vi "promień_krzywizny_pionowy.vi"(3 "e^2":dbl, 4 "a":dbl, 5 "fi[rad]":dbl) -> (1 "Promien krzywizny równoleżnika":dbl)   [LabVIEW 2015, in "Biblioteka moduł map v3.lvlib" / "Konwersja wsp.lvlib" / "UTM.lvlib"]
uses:
  UTM.lvlib
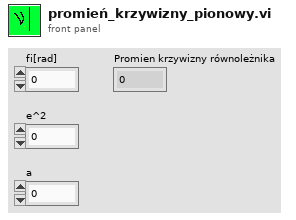
[diagram p1: front panel]
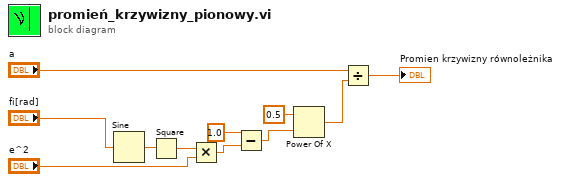
[diagram p0: block diagram]
diagram:
  n1 = Sine(x="fi[rad]") -> (sin(x)=w3:dbl)
  n2 = Square(x=w3) -> (x^2=w4:dbl)
  n3 = Multiply(x=w4, y="e^2") -> (x*y=w6:dbl)
  n4 = Subtract(x=1.0, y=w6) -> (x-y=w8:dbl)
  n5 = Power Of X(1:w8, 2:0.5 ("y")) -> (0:w10:dbl)
  n6 = Divide(x="a", y=w10) -> (x/y=→"Promien krzywizny równoleżnika":dbl)
